vi "Operational.vi"(8 "error in (no error)":errorcluster, 11 "Acquisition in":refnum<class "Acquisition.lvclass">) -> (0 "error out":errorcluster, 3 "Acquisition out":refnum<class "Acquisition.lvclass">)   [LabVIEW 2018, in "Acquisition.lvclass"]
uses:
  Acquisition.lvclass
  Acquisition.lvclass/Acquisition.ctl
  Server/Server.lvclass
  Channel/Channel.lvclass
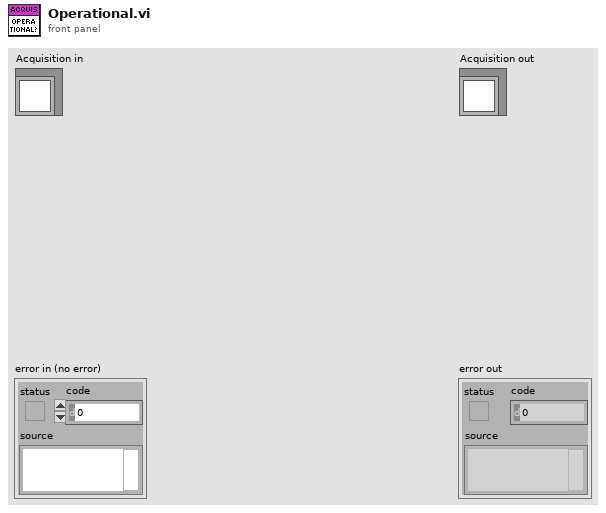
[diagram p1: front panel]
types:
  T1 = cluster{"Texp":dbl, "Nimages":u32, "InitialLine":u32, "FinalLine":u32, "InitialColumn":u32, "FinalColumn":u32, "EmGain":u32, "Cooler Off":bool, "CyclesDone":u32, "SequesDone":u32, "UsedDiskSpace":u16, "Error":bool}
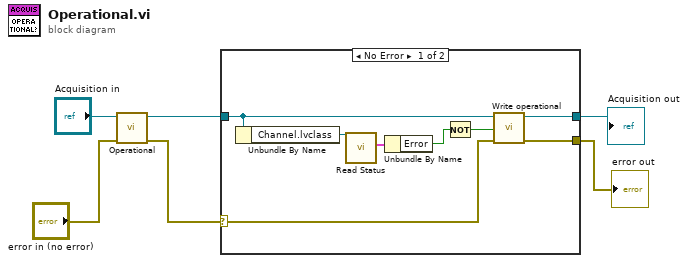
[diagram p0: block diagram]
diagram:
  n1 = call-parent "Operational.vi"("error in (no error)"="error in (no error)", "Server in"="Acquisition in") -> ("error out"=w4:errorcluster, "Server out"=w3:refnum<class "Acquisition.lvclass">)  [unwired: 8 in]
  n2 = case shown="No Error" w4 {
    selector: w4 -> [w9 w15]
    tunnel: w3 -> [w14 w16]
    tunnel: [w8 w15] -> w2
    tunnel: [w7 w16] -> w1
    frame No Error {
      n3 = Unbundle By Name(w14) -> ("Channel.lvclass"=w13:refnum<class "Channel.lvclass">)
      n4 = call-dynamic "Read Status.vi"("Channel in"=w13) -> ("Status"=w12:T1)  [unwired: 8 in, 2 out]
      n5 = Unbundle By Name(w12) -> ("Error"=w11:bool)
      n6 = Not(x=w11) -> (.not. x?=w10:bool)
      n7 = call-dynamic "Write operational.vi"("error in (no error)"=w9, "operational"=w10, "Server in"=w14) -> ("error out"=w8:errorcluster, "Server out"=w7:refnum<class "Acquisition.lvclass">)  [unwired: 7 in]
    }
    frame Error {
    }
  }
  "error out" <- w2
  "Acquisition out" <- w1
